vi "Enqueue SecondHandshake Connection.vi"(8 "Error In":errorcluster, 9 "Result":string, 10 "Barcode":string, 11 "Name":string) -> (0 "Error Out":errorcluster, 2 "Result":string)   [LabVIEW 2019, in "TCP2Foxconn.lvlib"]
uses:
  TCP2Foxconn.lvlib
  Queue/Queue.lvlib
  Data Error Notifier/Data and Error Notifier.lvlib
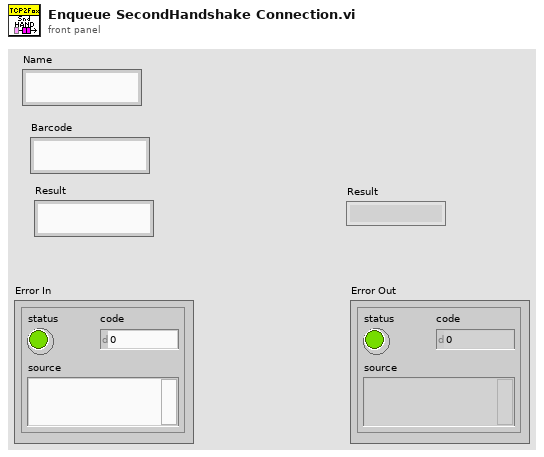
[diagram p1: front panel]
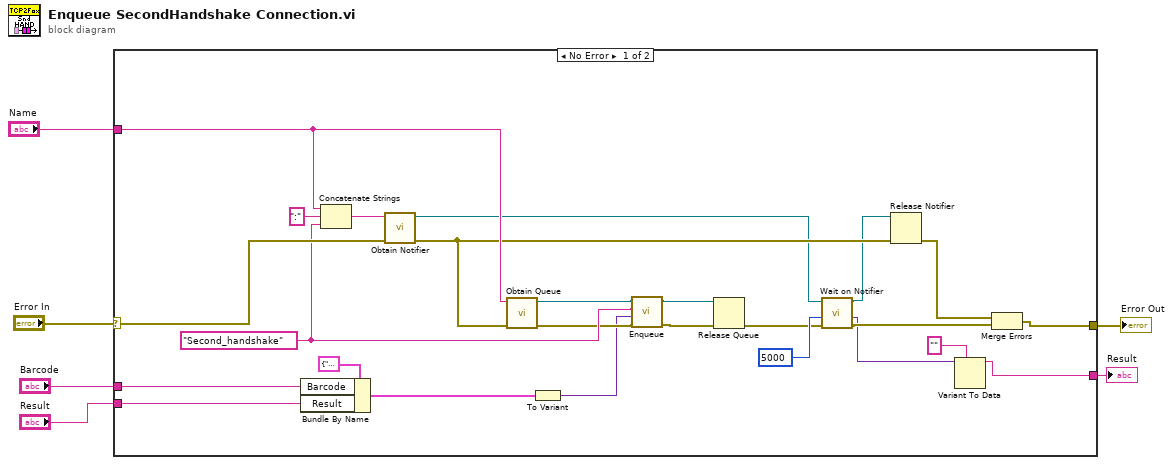
[diagram p0: block diagram]
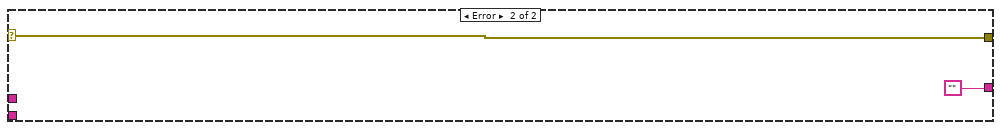
[diagram p2: hidden frame]
diagram:
  n1 = case shown="No Error" "Error In" {
    selector: "Error In" -> [w26 w33]
    tunnel: [w28 w33] -> w5
    tunnel: "Name" -> [w31 _]
    tunnel: [w13 ""] -> w2
    tunnel: "Barcode" -> [w9 _]
    tunnel: "Result" -> [w8 _]
    frame No Error {
      w23 = "Second_handshake" ("Message")
      n2 = Bundle By Name(cluster=cluster{"Barcode":string, "Result":string} {"Barcode"="", "Result"=""}, "Barcode"=w9, "Result"=w8) -> (w7:cluster{"Barcode":string, "Result":string})
      n3 = Concatenate Strings(w31, ":" ("string"), w23) -> (w27:string)
      n4 = call "Obtain Notifier.vi"("Error In"=w26, "Name"=w27) -> ("Error Out"=w25:errorcluster, "notifier out"=w19:refnum<notifier>)  [unwired: 8 in]
      n5 = call "Obtain Queue.vi"("Error In"=w25, "Name"=w31) -> ("Error Out"=w22:errorcluster, "queue out"=w24:refnum<queue>)  [unwired: 8 in]
      n6 = To Variant(anything=w7) -> (Variant=w12:variant)
      n7 = call "Enqueue.vi"("Error In"=w22, "Data"=w12, "Message"=w23, "queue in"=w24) -> ("Error Out"=w20:errorcluster, "queue out"=w21:refnum<queue>)  [unwired: 6 in]
      n8 = Release Queue(queue=w21, error in (no error)=w20) -> (error out=w17:errorcluster)  [unwired: 1 in, 2 out]
      n9 = call "Wait on Notifier.vi"("Error In"=w17, "timeout in ms (-1)"=5000, "notifier in"=w19) -> ("Error Out"=w15:errorcluster, "Data"=w14:variant, "notifier out"=w16:refnum<notifier>)  [unwired: 6 in]
      n10 = Release Notifier(notifier=w16, error in (no error)=w25) -> (error out=w29:errorcluster)  [unwired: 1 in, 2 out]
      n11 = Variant To Data(type="", Variant=w14) -> (data=w13:string)  [unwired: 1 in, 1 out]
      n12 = Merge Errors(w29, w15) -> (w28:errorcluster)
    }
    frame Error {
    }
  }
  "Error Out" <- w5
  "Result" <- w2
